vi "CANMOTORCONTROL.vi"() -> ()   [LabVIEW 2011]
panel:
  in  "Numeric":dbl
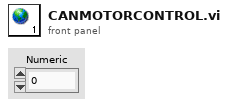
[diagram p1: front panel]
diagram:
